vi "F-Switch to Line.vi"() -> ()   [LabVIEW 2017]
uses:
  Support Code/Starting Position.ctl
panel:
  in  "Starting Position":T1
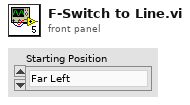
[diagram p1: front panel]
types:
  T1 = typedef "Starting Position.ctl" = enum16{"Far Left", "Center", "Far Right"}
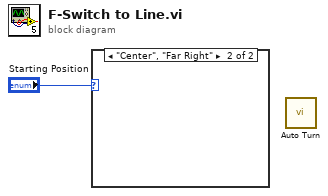
[diagram p0: block diagram]
diagram:
  n1 = case shown="\"Center\", \"Far Right\"" "Starting Position" {
    frame "Far Left", Default {
    }
    frame "Center", "Far Right" {
    }
  }
  n2 = call "Auto Turn.vi"() -> ()  [unwired: 11 in, 1 out]
